vi "User_Info.vi"(1 "String":string) -> ()   [LabVIEW 2010, in "FEMTO_LUCI-10.lvlib"]
uses:
  <userlib>/FEMTO/FEMTO_LUCI-10.lvlib
panel:
  in  "OK 2":bool
  # "Remote Control Operation"
  # "Remote Control Operation"
  # "Contact"
  # "FEMTO Messtechnik GmbH\n\nPhone:    +49-(0)30-280 4711-0\nemail:      info@femto.de\nWebsite:  www.femto.de"
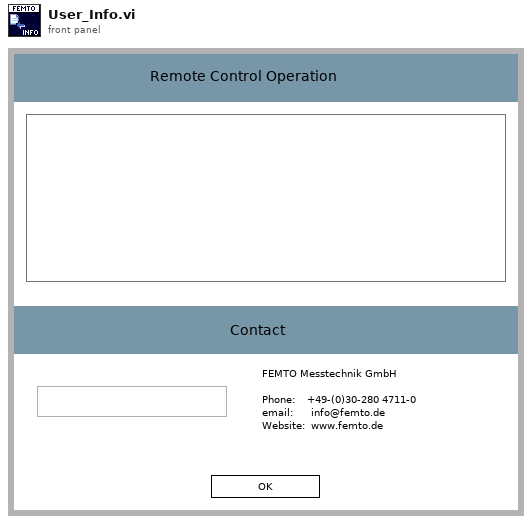
[diagram p1: front panel]
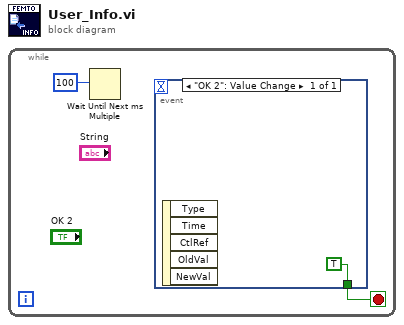
[diagram p0: block diagram]
diagram:
  n1 = while {
    stop <- w1 stop-if-true
    n2 = Wait Until Next ms Multiple(millisecond multiple=100) -> ()  [unwired: 1 out]
    n3 = event shown="[0] \"OK 2\": Value Change" {
      selector: _ -> [_]
      dyn-events: _ -> [_]
      timeout: _ -> [_]
      tunnel: [TRUE] -> w1
      event "OK 2": Value Change {
        n4 = event-data() -> ()  [unwired: 6 out]
      }
    }
  }
